vi "Init.vi"(8 "error in (no error)":errorcluster, 11 "Axsun_1310_SS in":refnum<class "Axsun_1310_SS.lvclass">) -> (0 "error out":errorcluster, 3 "Axsun_1310_SS out":refnum<class "Axsun_1310_SS.lvclass">)   [LabVIEW 2015, in "Axsun_1310_SS.lvclass"]
uses:
  Axsun_1310_SS.lvclass
  C:/Program Files (x86)/Axsun/Axsun OCT Control/AxsunOCTControl.dll
  Axsun_1310_SS.lvclass/Axsun_1310_SS.ctl
  Axsun VDL Global.vi
  Laser.lvclass
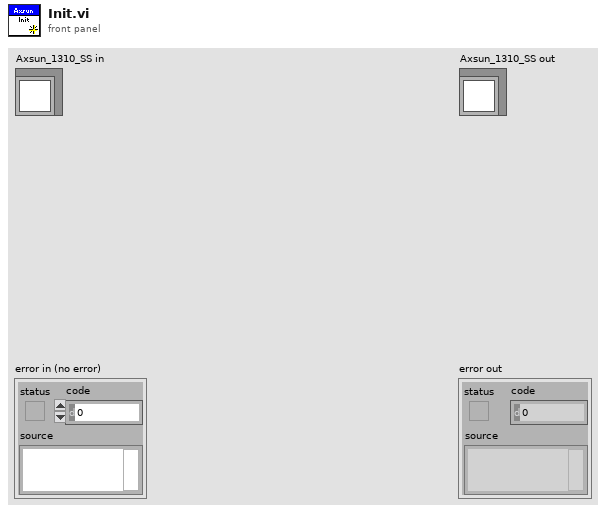
[diagram p1: front panel]
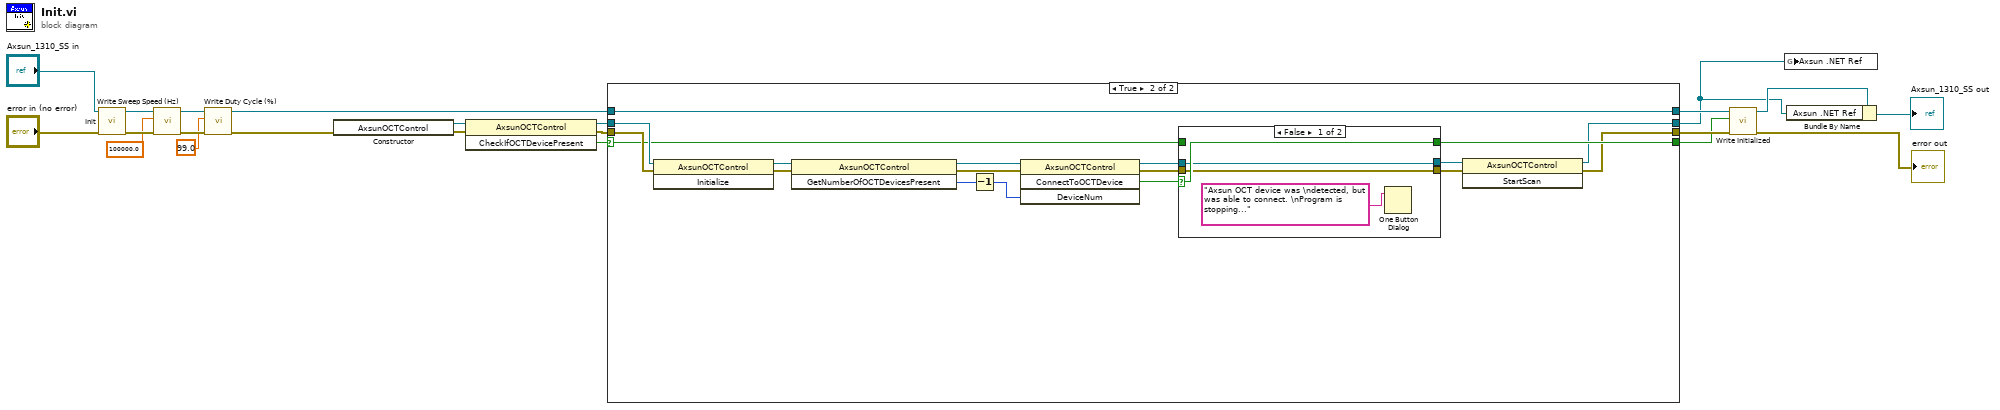
[diagram p0: block diagram]
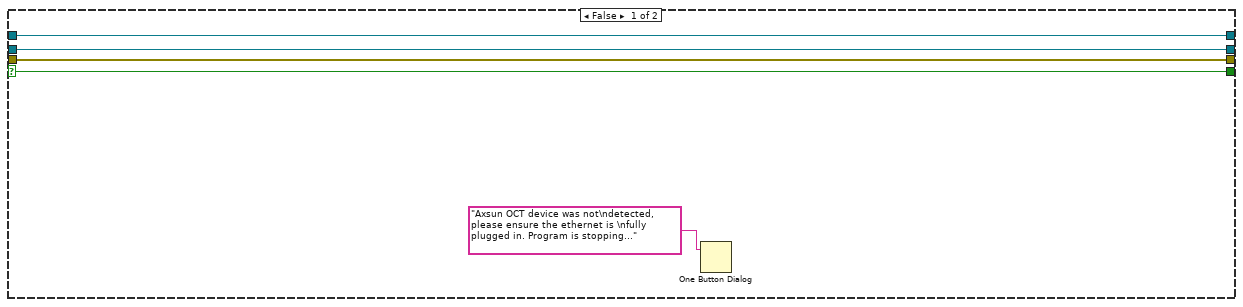
[diagram p2: hidden frame]
diagram:
  n1 = call-parent "Init.vi"("error in (no error)"="error in (no error)", "Laser in"="Axsun_1310_SS in") -> ("error out"=w8:errorcluster, "Laser out"=w9:refnum<class "Axsun_1310_SS.lvclass">)  [unwired: 8 in]
  n2 = call-dynamic "Write Sweep Speed (Hz).vi"("error in (no error)"=w8, "Sweep Speed (Hz)"=100000.0, "Laser in"=w9) -> ("error out"=w5:errorcluster, "Laser out"=w6:refnum<class "Axsun_1310_SS.lvclass">)  [unwired: 7 in]
  n3 = call-dynamic "Write Duty Cycle (%).vi"("error in (no error)"=w5, "Duty Cycle (%)"=99.0, "Laser in"=w6) -> ("error out"=w3:errorcluster, "Laser out"=w2:refnum<class "Axsun_1310_SS.lvclass">)  [unwired: 7 in]
  n4 = constructor class="AxsunOCTControl"(error in=w3) -> (reference out=w21:refnum<k24>, error out=w18:errorcluster)  [unwired: 2 in, 1 out]
  n5 = invoke class="AxsunOCTControl" method="CheckIfOCTDevicePresent"(reference=w21, error in=w18) -> (reference out=w19:refnum<k24>, error out=w16:errorcluster, "CheckIfOCTDevicePresent"=w17:bool)  [unwired: 1 in]
  n6 = case shown="True" w17 {
    selector: w17 -> [w26 w33]
    tunnel: w19 -> [w23 w44]
    tunnel: [w26 w32] -> w14
    tunnel: [w25 w28] -> w15
    tunnel: w16 -> [w25 w43]
    tunnel: w2 -> [w24 w45]
    tunnel: [w24 w45] -> w13
    tunnel: [w23 w29] -> w1
    frame False {
      n7 = One Button Dialog(message="Axsun OCT device was not\ndetected, please ensure the ethernet is \nfully plugged in. Program is stopping...") -> ()  [unwired: 1 in, 1 out]
    }
    frame True {
      n8 = invoke class="AxsunOCTControl" method="Initialize"(reference=w44, error in=w43) -> (reference out=w42:refnum<k24>, error out=w41:errorcluster)  [unwired: 1 in, 1 out]
      n9 = invoke class="AxsunOCTControl" method="GetNumberOfOCTDevicesPresent"(reference=w42, error in=w41) -> (reference out=w37:refnum<k24>, error out=w38:errorcluster, "GetNumberOfOCTDevicesPresent"=w40:i32)  [unwired: 1 in]
      n10 = Decrement(x=w40) -> (x-1=w39:i32)
      n11 = invoke class="AxsunOCTControl" method="ConnectToOCTDevice"(reference=w37, error in=w38, "DeviceNum"=w39) -> (reference out=w34:refnum<k24>, error out=w35:errorcluster, "ConnectToOCTDevice"=w36:bool)  [unwired: 1 in, 1 out]
      n12 = case shown="False" w36 {
        selector: w36 -> [w49 w52]
        tunnel: w35 -> [w47 w51]
        tunnel: w34 -> [w46 w50]
        tunnel: w33 -> [_ _]
        tunnel: [w49 w52] -> w32
        tunnel: [w47 w51] -> w30
        tunnel: [w46 w50] -> w31
        frame False {
          n13 = One Button Dialog(message="Axsun OCT device was \ndetected, but was able to connect. \nProgram is stopping...") -> ()  [unwired: 1 in, 1 out]
        }
        frame True {
          # "Do nothing"
        }
      }
      n14 = invoke class="AxsunOCTControl" method="StartScan"(reference=w31, error in=w30) -> (reference out=w29:refnum<k24>, error out=w28:errorcluster)  [unwired: 1 in, 1 out]
    }
  }
  n15 = call-dynamic "Write Initialized.vi"("error in (no error)"=w15, "Initialized"=w14, "Laser in"=w13) -> ("error out"=→"error out":errorcluster, "Laser out"=w12:refnum<class "Axsun_1310_SS.lvclass">)  [unwired: 7 in]
  n16 = global write "Axsun VDL Global.vi" "Axsun .NET Ref"(w1) -> ()
  n17 = Bundle By Name(cluster=w12, "Axsun .NET Ref"=w1) -> (→"Axsun_1310_SS out":refnum<class "Axsun_1310_SS.lvclass">)
